vi "8.2.-Momento Invariante de Hu Central - Upq.vi"(1 "q":dbl, 2 "p":dbl, 3 "X' Y'":dbl[](array[numeric]), 4 "f(x,y)":dbl[][](array[numeric])) -> (0 "Upq":dbl)   [LabVIEW 2020]
panel:
  # "Visión Artificial - Momentos Invariantes de Hu\nDiego Cervantes Rodríguez\ndicer0.com"
  # "Momento central = Upq = sum(sum(((X-xc)^p)*((Y-yc)^q)*f(x,y)))"
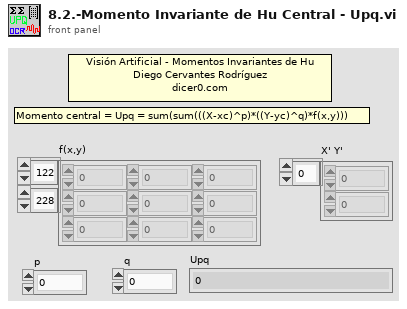
[diagram p1: front panel]
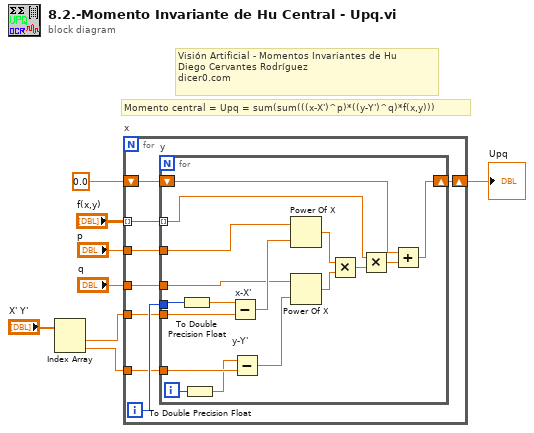
[diagram p0: block diagram]
diagram:
  # "Visión Artificial - Momentos Invariantes de Hu\nDiego Cervantes Rodríguez\ndicer0.com"
  # "Momento central = Upq = sum(sum(((x-X')^p)*((y-Y')^q)*f(x,y)))"
  n1 = Index Array "Index Array"(array="X' Y'") -> (element #1=w2:dbl, element #2=w1:dbl)  [unwired: 2 in]
  n2 = for "x" {
    tunnel: "f(x,y)" -> [w16] mode=indexing
    shift-right: [w15] -> w7
    shift-left: 0.0 -> [w14]
    tunnel: w2 -> [w12]
    tunnel: w1 -> [w11]
    tunnel: "p" -> [w10]
    tunnel: "q" -> [w9]
    i -> [w13]
    n3 = for "y" {
      tunnel: w16 -> [w20] mode=indexing
      shift-right: [w33] -> w15
      shift-left: w14 -> [w18]
      tunnel: w13 -> [w24]
      tunnel: w12 -> [w32]
      tunnel: w11 -> [w31]
      tunnel: w10 -> [w29]
      tunnel: w9 -> [w28]
      i -> [w26]
      n4 = To Double Precision Float(number=w24) -> (double precision float=w23:dbl)
      n5 = To Double Precision Float(number=w26) -> (double precision float=w25:dbl)
      n6 = Subtract "x-X'"(x=w23, y=w32) -> (x-y=w30:dbl)
      n7 = Subtract "y-Y'"(x=w25, y=w31) -> (x-y=w27:dbl)
      n8 = Power Of X(1:w30, 2:w29) -> (0:w22:dbl)
      n9 = Power Of X(1:w27, 2:w28) -> (0:w21:dbl)
      n10 = Multiply(x=w22, y=w21) -> (x*y=w19:dbl)
      n11 = Multiply(x=w20, y=w19) -> (x*y=w17:dbl)
      n12 = Add(x=w18, y=w17) -> (x+y=w33:dbl)
    }
  }
  "Upq" <- w7
